vi "test.vi"() -> ()   [LabVIEW 2023]
panel:
  out "2D Picture":picture
  out "Numeric":i32
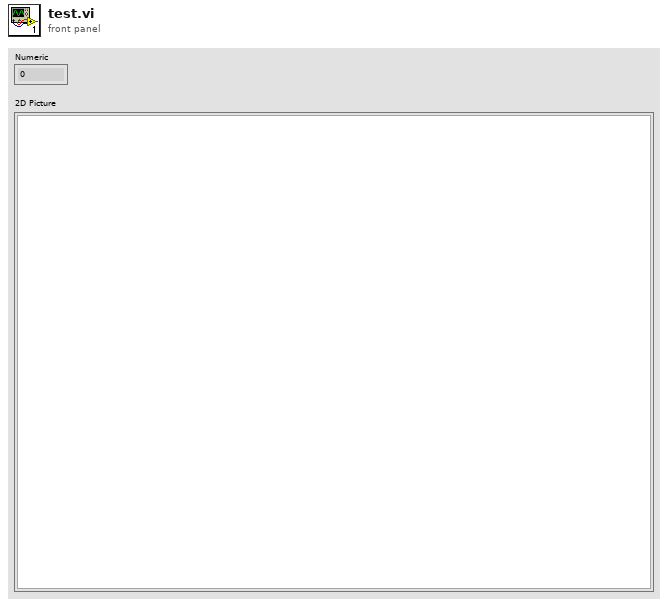
[diagram p1: front panel]
types:
  T1 = typedef "imagedata.ctl" = cluster{"image type":i32, "image depth":i32, "image":u8[], "mask":u8[], "colors":u32[], "Rectangle":cluster{"left":i16, "top":i16, "right":i16, "bottom":i16}}
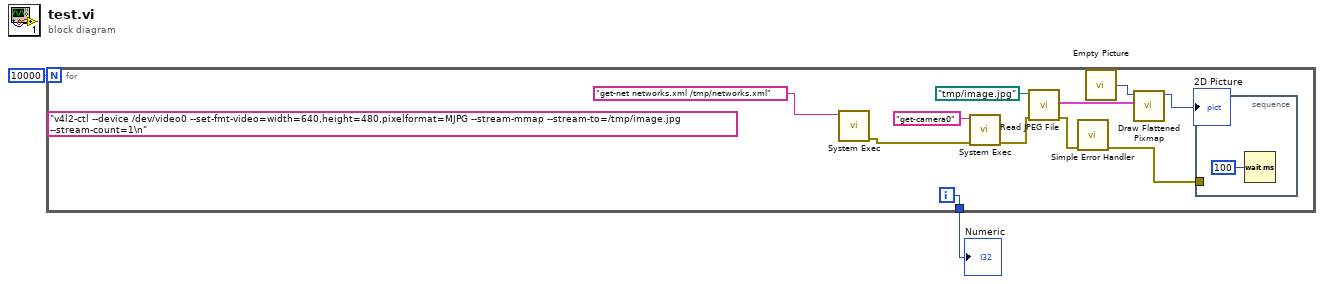
[diagram p0: block diagram]
diagram:
  n1 = for {
    N: 10000 -> [_]
    tunnel: [w5] -> w1
    i -> [w5]
    (unwired) "v4l2-ctl --device /dev/video0 --set-fmt-video=width=640,height=480,pixelformat=MJPG --stream-mmap --stream-to=/tmp/image.jpg --stream-count=1\n" ("command line")
    n2 = call <vilib>:"System Exec.vi"("command line"="get-net networks.xml /tmp/networks.xml" ("standard input")) -> ("error out"=w4:errorcluster)  [unwired: 7 in, 3 out]
    n3 = call <vilib>:"System Exec.vi"("error in (no error)"=w4, "command line"="get-camera0") -> ("error out"=w7:errorcluster)  [unwired: 6 in, 3 out]
    n4 = call <vilib>:"Read JPEG File.vi"("error in (no error)"=w7, "path to JPEG file"=path "/tmp/image.jpg") -> ("error out"=w9:errorcluster, "image data"=w13:T1)  [unwired: 7 in, 1 out]
    n5 = call <vilib>:"Simple Error Handler.vi"("error in (no error)"=w9) -> ("error out"=w8:errorcluster)  [unwired: 4 in, 4 out]
    n6 = call "Empty Picture"() -> ("empty picture"=w12:picture)
    n7 = call <vilib>:"Draw Flattened Pixmap.vi"("image data"=w13, "picture"=w12) -> ("new picture"=→"2D Picture":picture)  [unwired: 7 in]
    n8 = stacked-sequence {
      tunnel: w8 -> [_]
      frame #0 {
        n9 = Wait (ms)(milliseconds to wait=u32 100) -> ()  [unwired: 1 out]
      }
    }
  }
  "Numeric" <- w1
